vi "Decode Palette Description.vi"(8 "error in":errorcluster, 11 "Palette Description":string) -> (0 "error out":errorcluster, 1 "Inverted":string, 2 "Interpolated":string, 3 "# Colors":i32, 5 "Palette Name":string)   [LabVIEW 2021, in "Palette.lvlib"]
uses:
  Palette.lvlib
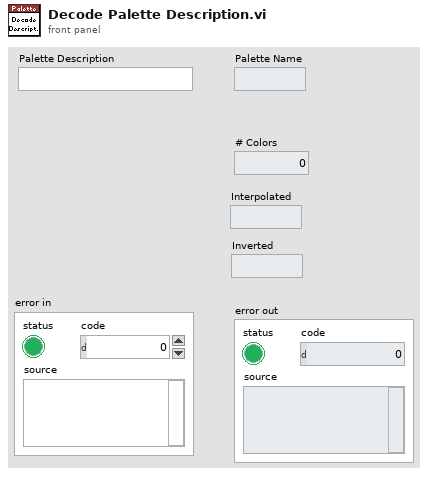
[diagram p1: front panel]
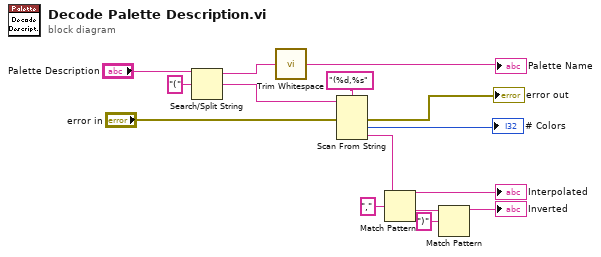
[diagram p0: block diagram]
diagram:
  n1 = Search/Split String(string="Palette Description", search string/char (-)="(") -> (substring before match=w4:string, match + rest of string=w5:string)  [unwired: 1 in, 1 out]
  n2 = call <vilib>:"Trim Whitespace.vi"("string"=w4) -> ("trimmed string"=→"Palette Name":string)  [unwired: 1 in]
  n3 = Scan From String(format string="(%d,%s", input string=w5, error in="error in") -> (error out=→"error out":errorcluster, output 1=→"# Colors":i32, output 2=w2:string)  [unwired: 3 in, 2 out]
  n4 = Match Pattern(string=w2, regular expression=",") -> (before substring=→"Interpolated":string, after substring=w14:string)  [unwired: 1 in, 2 out]
  n5 = Match Pattern(string=w14, regular expression=")") -> (before substring=→"Inverted":string)  [unwired: 1 in, 3 out]
